vi "PH_SM_Class.contents.vi"   [LabVIEW 2014, in "PH_SM_Class.lvlib"]
doc: "This class is forseen to collect data of PHELIX devices around a PHELIX shot. It uses the ReadData-Method and stores the data in LabVIEW format. They can be visualized using the class PH_DataViewer. \n\nThis class is part of the PHELIX application layer."
uses:
  PH_SM_Class.lvlib
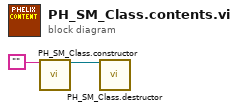
[diagram p0: block diagram]
diagram:
  n1 = call "PH_SM_Class.constructor.vi"("name"="") -> ("i ref out"=w1:refnum<vi>)  [unwired: 16 in, 2 out]
  n2 = call "PH_SM_Class.destructor.vi"("i ref in"=w1) -> ()  [unwired: 18 in, 1 out]
